vi "p1.vi"() -> ()   [LabVIEW 2021, in "d19.lvlib"]
uses:
  d19.lvlib
  Blueprint/Blueprint.lvclass
  Blueprint/Blueprint.lvclass/Blueprint.ctl
  Mine/Schedule Ore Robot.vi
  Mine/Schedule Clay Robot.vi
  Mine/Schedule Obsidian Robot.vi
  Mine/Schedule Geode Robot.vi
  AOC/AOC.lvlib
panel:
  in  "Choice":i32[](array[numeric])
  in  "Max Time":u8=24
  out "Quality Level":i32=30
  out "Geodes":u8=1
  out "Blueprint":i32=1
  in  "Example":string="Blueprint 1:  Each ore robot costs 4 ore.  Each clay robot costs 2 ore.  Each obsidian robot costs 3 ore and 14 clay.  Each geode robot costs 2 ore and 7 obsidian.\nBlueprint 2:  Each ore robot costs 2 ore.  Each clay robot costs 3 ore.  Each obsidian robot costs 3 ore and 8 clay.  Each geode robot costs 3 ore and 12 obsidian."
  in  "Example":bool=TRUE
  out "Answer":i32=978
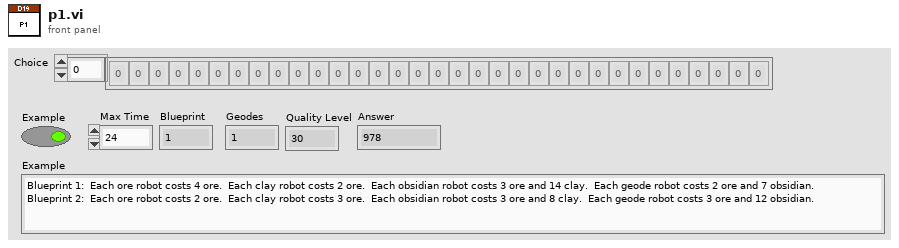
[diagram p1: front panel]
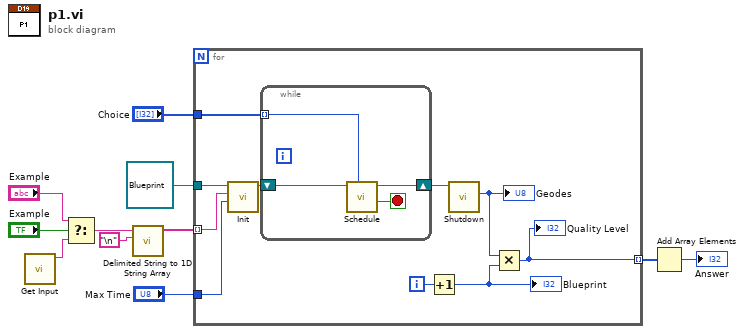
[diagram p0: block diagram]
diagram:
  n1 = call "Get Input.vi"() -> ("Input"=w11:string)  [unwired: 11 in]
  n2 = Select(t="Example", s="Example", f=w11) -> (s? t:f=w10:string)
  n3 = call <vilib>:"Delimited String to 1D String Array.vi"("delimiter"="\n", "delimited string"=w10) -> ("string array"=w6:string[])  [unwired: 9 in]
  n4 = for {
    tunnel: w6 -> [w21] mode=indexing
    tunnel: refnum<class "Blueprint.lvclass"> refnum ("Bluepriny in") -> [w19]
    tunnel: [w17] -> w4 mode=indexing
    tunnel: "Max Time" -> [w16]
    tunnel: "Choice" -> [w12]
    i -> [w20]
    n5 = call "Init.vi"("Max Time"=w16, "Blueprint String"=w21, "Blueprint in"=w19) -> ("Blueprint out"=w15:refnum<class "Blueprint.lvclass">)  [unwired: 8 in]
    n6 = while {
      shift-right: [w23] -> w14
      shift-left: w15 -> [w24]
      tunnel: w12 -> [w22] mode=indexing
      stop <- w25 stop-if-true
      n7 = call "Schedule.vi"("Choice"=w22, "Blueprint in"=w24) -> ("Finished?"=w25:bool, "Blueprint out"=w23:refnum<class "Blueprint.lvclass">)  [unwired: 7 in, 1 out]
    }
    n8 = Increment(x=w20) -> (x+1=w18:i32)
    "Blueprint" <- w18
    n9 = call "Shutdown.vi"("Blueprint in"=w14) -> ("max geodes"=w13:u8)  [unwired: 9 in, 1 out]
    "Geodes" <- w13
    n10 = Multiply(x=w13, y=w18) -> (x*y=w17:i32)
    "Quality Level" <- w17
  }
  n11 = Add Array Elements(numeric array=w4) -> (sum=→"Answer":i32)
